vi "Stop Laser.vi"(8 "error in (no error)":errorcluster, 11 "Laser Controller API in":refnum<class "Laser Controller.lvclass">) -> (0 "error out":errorcluster, 3 "Laser Controller API out":refnum<class "Laser Controller.lvclass">)   [LabVIEW 2022 SP3, in "Laser Controller.lvclass"]
uses:
  Laser Controller.lvclass
  Laser Controller.lvclass/Laser Controller.ctl
  XY Stage/Process Actor/Process Framework/Process State Data/Process State Data.lvclass/Process State Data.ctl
  XY Stage/Process Actor/Process Framework/Interlock Q Class/Interlock Q Class.lvclass/Interlock Q Class.ctl
  <vilib>/ActorFramework/Message Enqueuer/Message Enqueuer.lvclass/Message Enqueuer.ctl
  XY Stage/Process Actor/Process Framework/Process State Data/Accessor/Write Abort.vi
  <vilib>/ActorFramework/Message Enqueuer/Enqueue.vi
  XY Stage/Process Actor/Process Framework/Interlock Q Class/Accessor/Read Process Q.vi
  Laser Process/Laser Process Messages/Stop Laser Msg/Stop Laser Msg.lvclass
  C:/Program Files/National Instruments/LabVIEW 2022/vi.lib/ActorFramework/Message/Message.lvclass
  <vilib>/ActorFramework/Message Priority Queue/Priority Enqueue.vi
  <vilib>/ActorFramework/Message Enqueuer/Message Enqueuer.lvclass
  XY Stage/Process Actor/Process Framework/Process State Data/Process State Data.lvclass
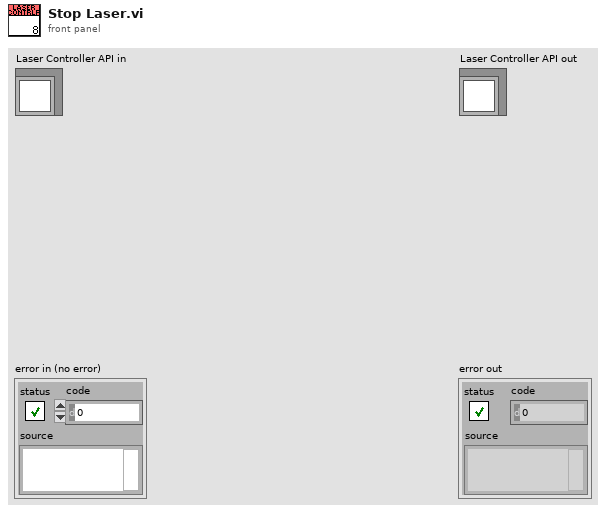
[diagram p1: front panel]
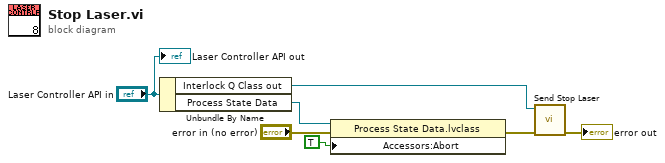
[diagram p0: block diagram]
diagram:
  n1 = Unbundle By Name("Laser Controller API in") -> ("Interlock Q Class out"=w1:refnum<class "Interlock Q Class.lvclass">, "Process State Data"=w5:refnum<data-value>)
  n2 = property class="Process State Data.lvclass"(reference=w5, error in="error in (no error)", "Accessors:Abort"=TRUE ("Abort")) -> (error out=w2:errorcluster)  [unwired: 1 out]
  n3 = call "Send Stop Laser.vi"("error in (no error)"=w2, "Interlock Q Class"=w1) -> ("error out"=→"error out":errorcluster)  [unwired: 8 in, 1 out]
  "Laser Controller API out" <- "Laser Controller API in"
